vi "SpatialDual_Messenger.vi"(7 "Queue in":refnum<queue>, 10 "Time Out":bool) -> ()   [LabVIEW 2019]
uses:
  Globals and Definitions/System Message.ctl
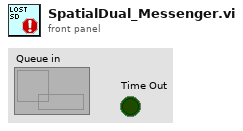
[diagram p1: front panel]
types:
  T1 = typedef "System Message.ctl" = cluster{"Message Tag":string, "Message Body":string, "Snooze Time (s)":dbl, "Snooze Alert?":bool, "Log Event?":bool, "Send Email":i32}
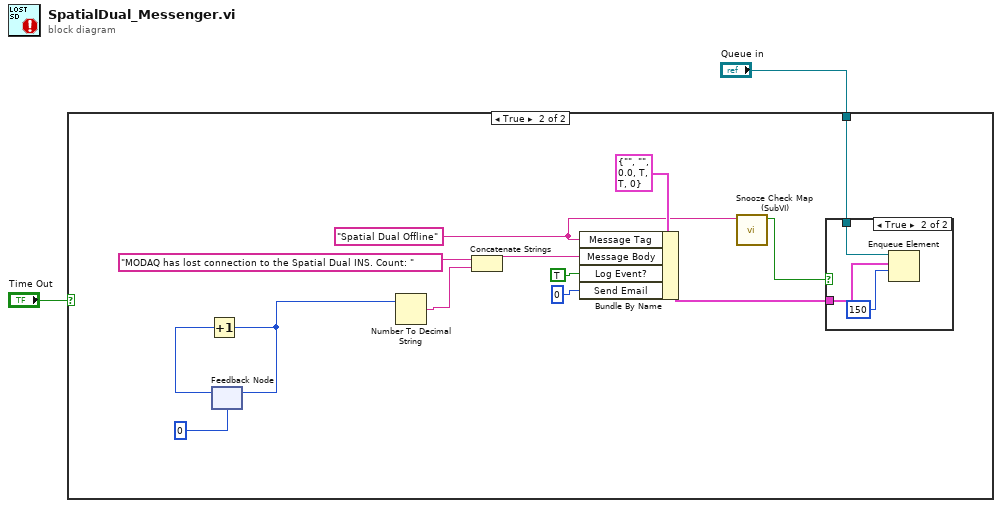
[diagram p0: block diagram]
diagram:
  n1 = case shown="True" "Time Out" {
    tunnel: "Queue in" -> [_ w7]
    frame False {
    }
    frame True {
      w9 = "Spatial Dual Offline" ("Message Tag")
      n2 = feedback #1(0) -> (w11:i32)
      n3 = Increment(x=w11) -> (x+1=w6:i32)
      n4 = feedback-in #1(w6) -> ()
      n5 = Number To Decimal String(number=w6) -> (decimal integer string=w3:string)  [unwired: 1 in]
      n6 = Concatenate Strings("MODAQ has lost connection to the Spatial Dual INS. Count: " ("Message Body"), w3) -> (w5:string)
      n7 = Bundle By Name(cluster=T1 {"Message Tag"="", "Message Body"="", "Snooze Time (s)"=0.0, "Snooze Alert?"=TRUE, "Log Event?"=TRUE, "Send Email"=0}, "Message Tag"=w9, "Message Body"=w5, "Log Event?"=TRUE, "Send Email"=0) -> (w14:T1)
      n8 = call "Snooze Check Map (SubVI).vi"("key"=w9) -> ("Snooze Expired?"=w8:bool)  [unwired: 10 in]
      n9 = case shown="True" w8 {
        tunnel: w14 -> [_ w17]
        tunnel: w7 -> [_ w18]
        frame False {
        }
        frame True {
          n10 = Enqueue Element(queue=w18, element=w17, timeout in ms (-1)=150) -> ()  [unwired: 1 in, 3 out]
        }
      }
    }
  }
